vi "get desired keys.vi"(8 "error in":errorcluster, 11 "AppStateMachine configuration in":refnum<class "AppStateMachine configuration.lvclass">) -> (0 "error out":errorcluster, 2 "desired keys":string[](array[string]), 3 "AppStateMachine configuration out":refnum<class "AppStateMachine configuration.lvclass">)   [LabVIEW 2017, in "AppStateMachine configuration.lvclass"]
uses:
  AppStateMachine configuration.lvclass
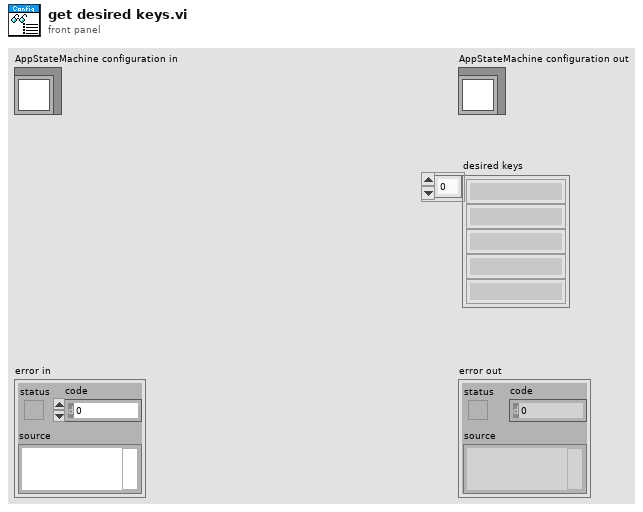
[diagram p1: front panel]
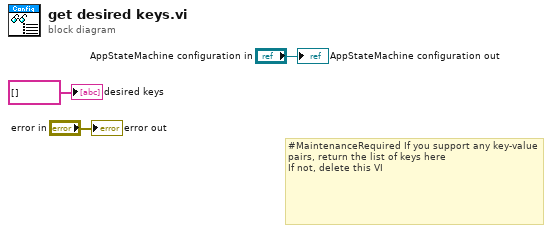
[diagram p0: block diagram]
diagram:
  # "#MaintenanceRequired If you support any key-value pairs, return the list of keys here\nIf not, delete this VI"
  "error out" <- "error in"
  "AppStateMachine configuration out" <- "AppStateMachine configuration in"
  "desired keys" <- string[] [] ("desired keys")
